vi "FlatToRichsift_proxy_v1_IngestDataStreamStringRequest.vi"(5 "OutputClusterType":T1, 11 "InputCluster":T3) -> (3 "OutputCluster":T1)   [LabVIEW 2024, in "SiftProxy_client.lvlib"]
uses:
  sift_proxy_v1_IngestDataStreamStringRequest_Flat.ctl
  google_protobuf_Timestamp_Flat.ctl
  sift_proxy_v1_IngestDataStreamStringRequest.ctl
  google_protobuf_Timestamp.ctl
  SiftProxy_client.lvlib
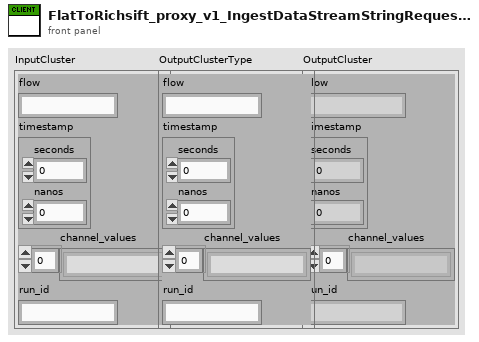
[diagram p1: front panel]
types:
  T1 = typedef "SiftProxy_client.lvlib/sift_proxy_v1_IngestDataStreamStringRequest.ctl" = cluster{"flow":string, "timestamp":T2, "channel_values":string[], "run_id":string}
  T2 = typedef "SiftProxy_client.lvlib/google_protobuf_Timestamp.ctl" = cluster{"seconds":i64, "nanos":i32}
  T3 = typedef "SiftProxy_client.lvlib/sift_proxy_v1_IngestDataStreamStringRequest_Flat.ctl" = cluster{"flow":string, "timestamp":T4, "channel_values":string[], "run_id":string}
  T4 = typedef "SiftProxy_client.lvlib/google_protobuf_Timestamp_Flat.ctl" = cluster{"seconds":i64, "nanos":i32}
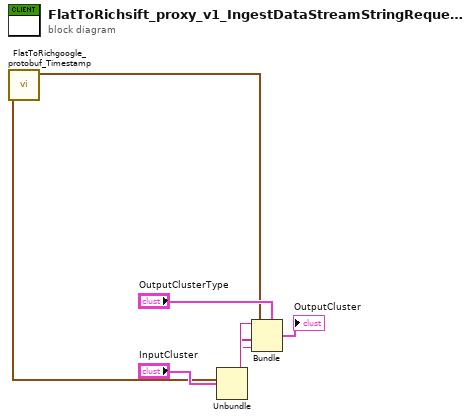
[diagram p0: block diagram]
diagram:
  n1 = Unbundle "Unbundle"("InputCluster") -> ("flow"=w5:string, "timestamp"=w4:T4, "channel_values"=w2:string[], "run_id"=w1:string)
  n2 = call "FlatToRichgoogle_protobuf_Timestamp.vi"("InputCluster"=w4) -> ("OutputCluster"=w3:T2)  [unwired: 10 in]
  n3 = Bundle "Bundle"(cluster="OutputClusterType", "flow"=w5, "timestamp"=w3, "channel_values"=w2, "run_id"=w1) -> (→"OutputCluster":T1)
